vi "LeapMain.vi"() -> ()   [LabVIEW 2017]
uses:
  LeapMotion/TypeDefs/SelectSign.ctl
  LeapMotion/TypeDefs/StateSelector.ctl
  MachineLearning/TypeDefs/Label Setting.ctl
  C:/Users/snordinh/Desktop/LEAP-sign-language-test/LEAP-sign-language-test/LeapMotion/Dynamic Libraries/LeapCSharp.NET4.5.dll
  LeapMotion/Dynamic Libraries/LeapCSharp.NET4.5.dll
  LeapMotion/LeapMotion.lvlib
  MachineLearning/MachineLearning.lvlib
panel:
  in  "Clear text":bool
  in  "Interpret hand sign":bool
  out "Interpreted text":string
  in  "Tab Control":T1(tab)
  out "Real-time plot":cluster{sgl[], sgl[]}[](graph)
  out "Detected hand sign":T2
  out "feature trend deployment":dbl[][](graph)
  out "predicted result":i32[][](graph)
  out "metrics":T3
  in  "Error In":errorcluster
  out "Error out":errorcluster
  in  "Trained ML model":path=path "C:/Users/snordinh/Desktop/LEAP-sign-language-test/LEAP-sign-language-test/MachineLearning/SubVIs/WithDan.json"
  in  "Save model as":path
  in  "Train model":bool
  out "Points left to log":i32
  in  "Start logging":bool
  out "File saved as":path
  in  "Write header":bool
  in  "Points per sign":i32=100
  out "feature trend training":dbl[][](graph)
  out "Left hand detected":bool
  out "Right hand detected":bool
  in  "Hand sign":T2
  in  "Stop Program":bool
  out "LEAP connected?":bool
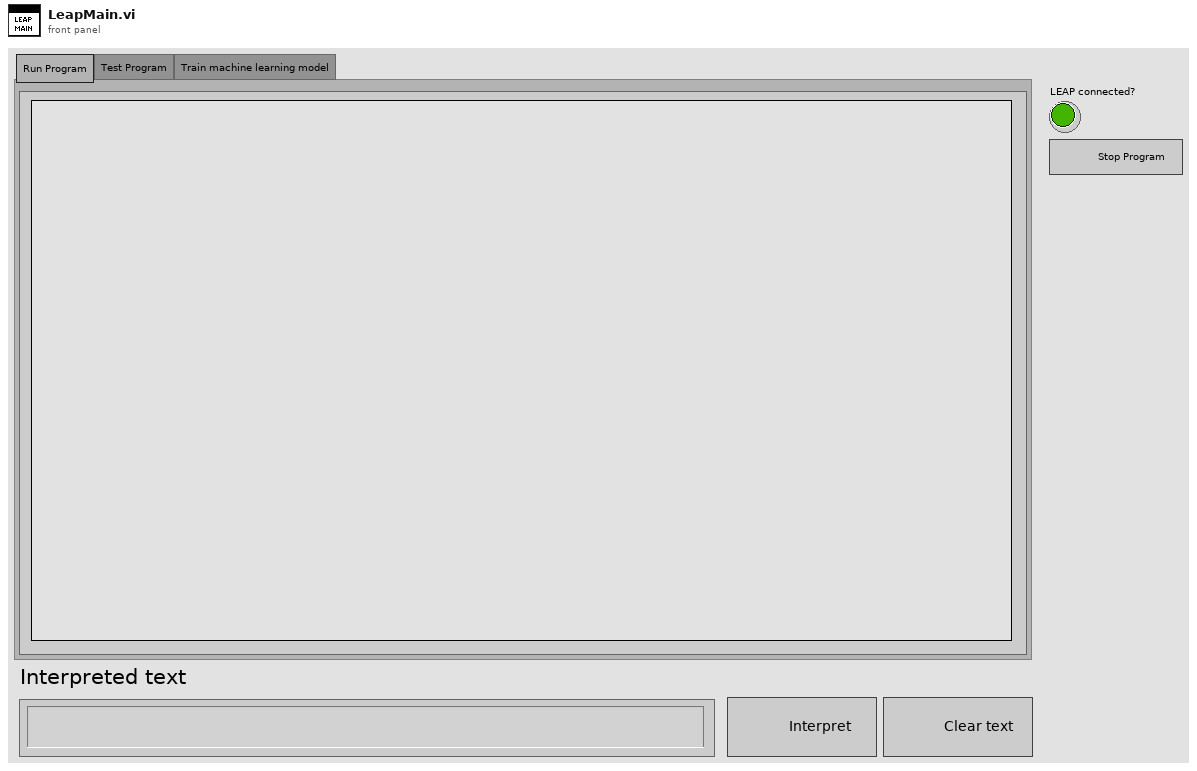
[diagram p1: front panel]
types:
  T1 = enum32{"Run Program", "Test Program", "Train machine learning model"}
  T2 = typedef "LeapMotion.lvlib/SelectSign.ctl" = enum16{"A", "B", "C", "D", "E", "F", "G", "H", "I", "J", "K", "L", "M", "N", "O", "P", "Q", "R", "S", "T", "U", "V", "W", "X", "Y", "Z"}
  T3 = cluster{"accuracy":dbl, "precision":dbl, "recall":dbl, "f1 score":dbl}
  T4 = typedef "LeapMotion.lvlib/StateSelector.ctl" = enum16{"Initialize", "Display", "Logging sequence", "Train model", "Classify", "Write Header", "Stop"}
  T5 = typedef "MachineLearning.lvlib/Label Setting.ctl" = cluster{"with label column?":bool, "label column index":i32}
  T6 = typedef "LeapMotion.lvlib/LEAPframe.ctl" = cluster{"Id":i64, "Timestamp":i64, "CurrentFramesPerSecond":sgl, "Hands":T7[]}
  T7 = typedef "LeapMotion.lvlib/LEAPhand.ctl" = cluster{"IsLeft":bool, "IsRight":bool, "Id":i32, "FrameId":i64, "Confidence":sgl, "TimeVisible":sgl, "PalmPosition":T8, "Fingers":T9[]}
  T8 = typedef "LeapMotion.lvlib/LEAPvector.ctl" = cluster{"Pitch":sgl, "Yaw":sgl, "Roll":sgl, "Magnitude":sgl, "XYZ":sgl[]}
  T9 = typedef "LeapMotion.lvlib/LEAPfinger.ctl" = cluster{"IsExtended":bool, "Id":i32, "Type":i32, "HandId":i32, "Length":sgl, "Width":sgl, "TimeVisible":sgl, "TipPosition":T8, "Bones":T10[]}
  T10 = typedef "LeapMotion.lvlib/LEAPbone.ctl" = cluster{"Type":i32, "Width":sgl, "Length":sgl, "Center":T8, "Direction":T8, "NextJoint":T8, "PrevJoint":T8}
  T11 = enum16{"SVM", "Neural Network", "Logistic Regression"}
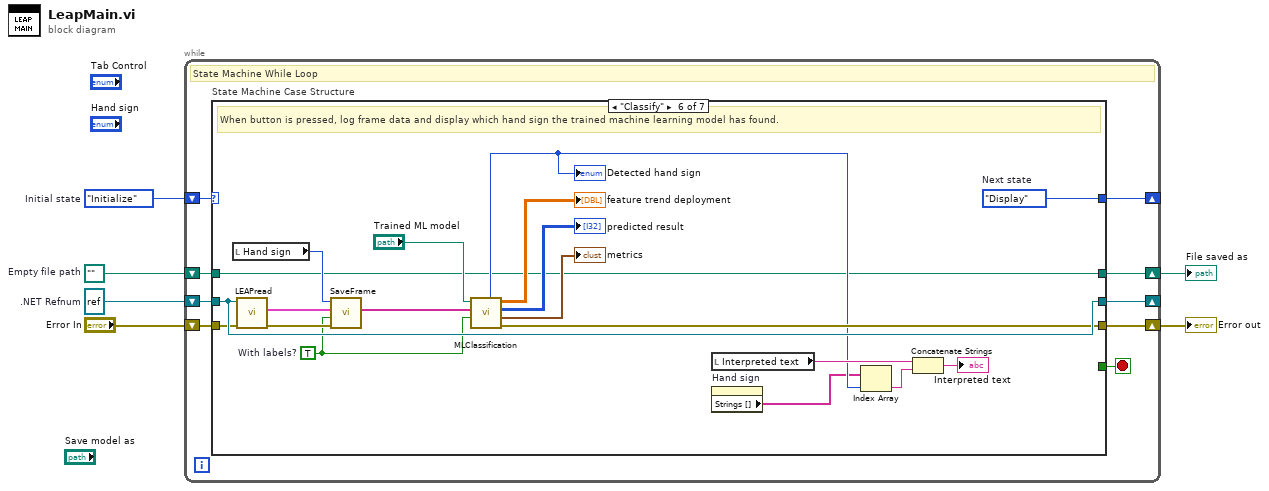
[diagram p0: block diagram]
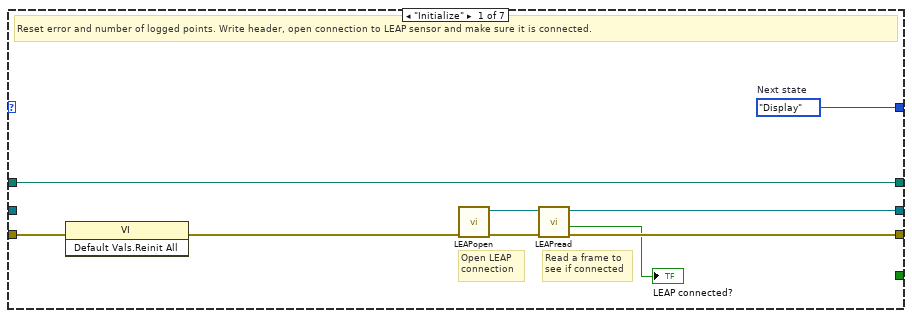
[diagram p2: hidden frame]
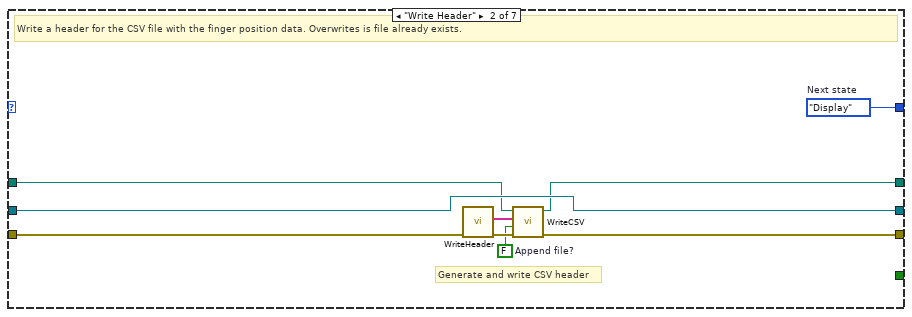
[diagram p3: hidden frame]
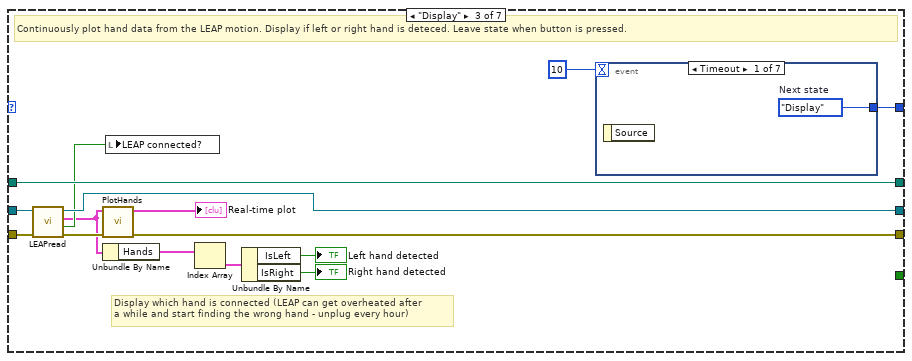
[diagram p4: hidden frame]
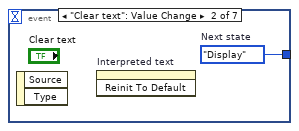
[diagram p5: hidden frame]
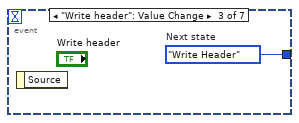
[diagram p6: hidden frame]
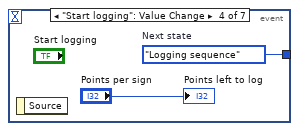
[diagram p7: hidden frame]
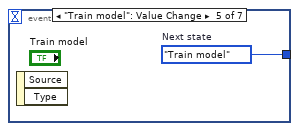
[diagram p8: hidden frame]
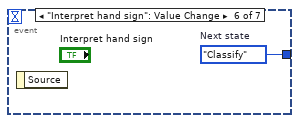
[diagram p9: hidden frame]
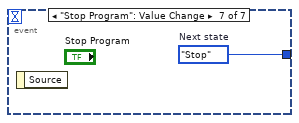
[diagram p10: hidden frame]
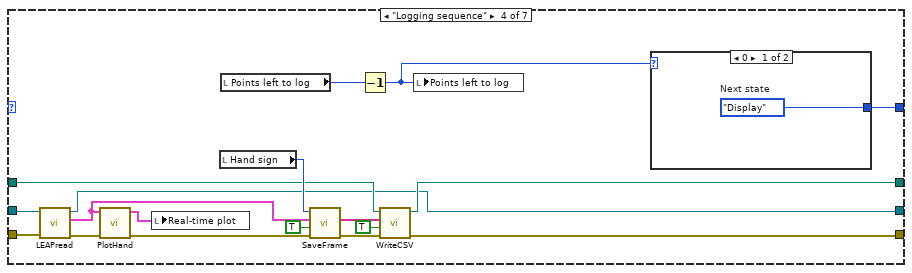
[diagram p11: hidden frame]
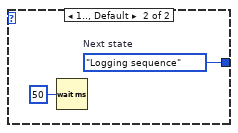
[diagram p12: hidden frame]
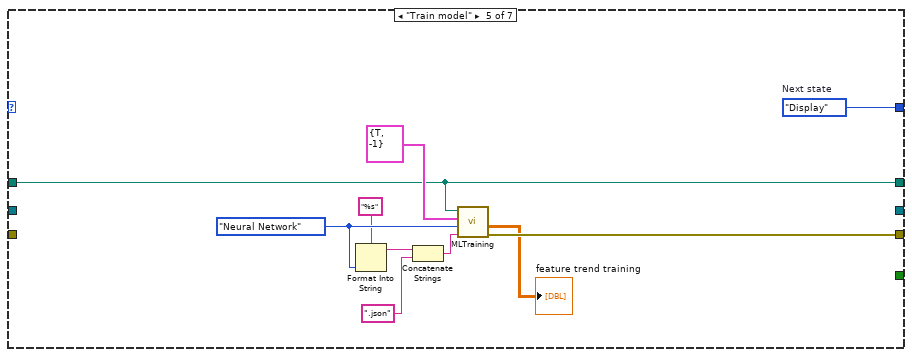
[diagram p13: hidden frame]
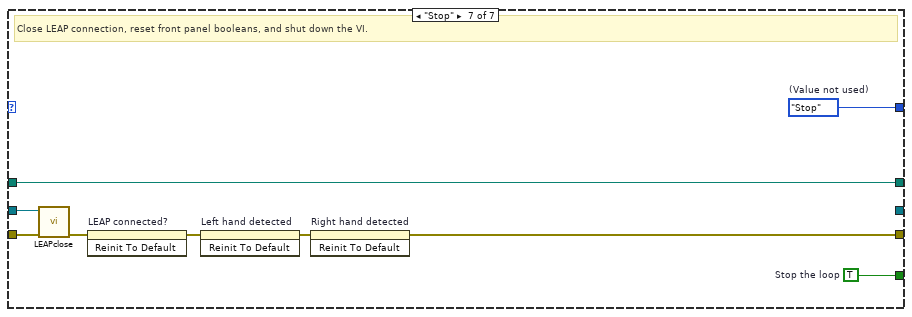
[diagram p14: hidden frame]
diagram:
  w4 = path ""  # Empty file path
  w2 = refnum<k24> refnum  # .NET Refnum
  w1 = StateSelector."Initialize"  # Initial state
  n1 = while {
    shift-right: [w15] -> _
    shift-left: w2 -> [w13]
    shift-right: [w14] -> w5
    shift-left: "Error In" -> [w12]
    shift-right: [w9] -> w3
    shift-left: w4 -> [w10]
    shift-right: [w7] -> _
    shift-left: w1 -> [w8]
    stop <- w11 stop-if-true
    # "State Machine While Loop"
    n2 = case "State Machine Case Structure" shown="\"Classify\"" w8 {
      tunnel: [_ _ _ _ _ _ w115] -> w11
      tunnel: [w17 w33 w40 w59 _ w103 _] -> w15
      tunnel: [w19 w27 w37 w60 w87 w96 w112] -> w14
      tunnel: w13 -> [_ w33 w42 w73 _ w103 w110]
      tunnel: w12 -> [w24 w32 w41 w74 _ w102 w109]
      tunnel: w10 -> [w23 w29 w43 w62 w84 w92 w111]
      tunnel: [w23 w28 w43 w61 w84 w92 w111] -> w9
      tunnel: [w16 w25 w34 w57 w79 w89 w107] -> w7
      frame "Initialize" {
        w16 = StateSelector."Display"  # Next state
        # "Read a frame to\nsee if connected"
        # "Open LEAP \nconnection"
        # "Reset error and number of logged points. Write header, open connection to LEAP sensor and make sure it is connected."
        n3 = invoke class="VI" method="Default Vals.Reinit All"(error in=w24) -> (error out=w22:errorcluster)  [unwired: 2 in, 2 out]
        n4 = call "LEAPopen.vi"("error in (no error)"=w22) -> ("error out"=w20:errorcluster, "Leap.Controller"=w21:refnum<k24>)  [unwired: 9 in]
        n5 = call "LEAPread.vi"("error in (no error)"=w20, "Controller Refnum In"=w21) -> ("error out"=w19:errorcluster, "IsConnected"=→"LEAP connected?":bool, "Leap.Controller"=w17:refnum<k24>)  [unwired: 6 in, 1 out]
      }
      frame "Write Header" {
        w26 = FALSE  # Append file?
        w25 = StateSelector."Display"  # Next state
        # "Generate and write CSV header"
        # "Write a header for the CSV file with the finger position data. Overwrites is file already exists."
        n6 = call "WriteHeader.vi"("Error in"=w32) -> ("Error out"=w31:errorcluster, "Header string array"=w30:string[])  [unwired: 9 in]
        n7 = call "WriteCSV.vi"("error in (no error)"=w31, "Append file?"=w26, "Data to write"=w30, "CSV file path in"=w29) -> ("error out"=w27:errorcluster, "CSV file path out"=w28:path)  [unwired: 6 in]
      }
      frame "Display" {
        # "Display which hand is connected (LEAP can get overheated after\na while and start finding the wrong hand - unplug every hour)"
        # "Continuously plot hand data from the LEAP motion. Display if left or right hand is deteced. Leave state when button is pressed."
        n8 = call "LEAPread.vi"("error in (no error)"=w41, "Controller Refnum In"=w42) -> ("error out"=w36:errorcluster, "IsConnected"=w39:bool, "Frame"=w35:T6, "Leap.Controller"=w40:refnum<k24>)  [unwired: 6 in]
        n9 = call "PlotHands.vi"("error in"=w36, "Frame"=w35) -> ("error out"=w37:errorcluster, "Data to plot"=→"Real-time plot":cluster{"Array":sgl[], "Array":sgl[]}[])  [unwired: 8 in]
        n10 = Unbundle By Name(w35) -> ("Hands"=w44:T7[])
        n11 = local write "LEAP connected?"(w39) -> ()
        n12 = Index Array(array=w44) -> (element=w45:T7)  [unwired: 1 in]
        n13 = Unbundle By Name(w45) -> ("IsLeft"=→"Left hand detected":bool, "IsRight"=→"Right hand detected":bool)
        n14 = event shown="[0] Timeout" {
          selector: _ -> [_ _ _ _ _ _ _]
          dyn-events: _ -> [_ _ _ _ _ _ _]
          timeout: 10 -> [_ _ _ _ _ _ _]
          tunnel: [w49 w50 w51 w53 w54 w55 w56] -> w34
          event Timeout {
            w49 = StateSelector."Display"  # Next state
            n15 = event-data() -> ()  [unwired: 1 in, 1 out]
          }
          event "Clear text": Value Change {
            w50 = StateSelector."Display"  # Next state
            n16 = event-data() -> ()  [unwired: 1 in, 2 out]
            n17 = invoke on="Interpreted text" class="Str" method="Reinit To Default"() -> ()  [unwired: 3 in, 3 out]
          }
          event "Write header": Value Change {
            w51 = StateSelector."Write Header"  # Next state
            n18 = event-data() -> ()  [unwired: 1 in, 1 out]
          }
          event "Start logging": Value Change {
            w53 = StateSelector."Logging sequence"  # Next state
            n19 = event-data() -> ()  [unwired: 1 in, 1 out]
            "Points left to log" <- "Points per sign"
          }
          event "Train model": Value Change {
            w54 = StateSelector."Train model"  # Next state
            n20 = event-data() -> ()  [unwired: 1 in, 2 out]
          }
          event "Interpret hand sign": Value Change {
            w55 = StateSelector."Classify"  # Next state
            n21 = event-data() -> ()  [unwired: 1 in, 1 out]
          }
          event "Stop Program": Value Change {
            w56 = StateSelector."Stop"  # Next state
            n22 = event-data() -> ()  [unwired: 1 in, 1 out]
          }
        }
      }
      frame "Logging sequence" {
        n23 = call "LEAPread.vi"("error in (no error)"=w74, "Controller Refnum In"=w73) -> ("error out"=w72:errorcluster, "Frame"=w67:T6, "Leap.Controller"=w59:refnum<k24>)  [unwired: 6 in, 1 out]
        n24 = call "PlotHand.vi"("error in"=w72, "Frame"=w67) -> ("error out"=w71:errorcluster, "Data to plot"=w68:cluster{"Array":sgl[], "Array":sgl[]}[])  [unwired: 8 in]
        n25 = local write "Real-time plot"(w68) -> ()
        n26 = local read "Hand sign"() -> (w69:T2)
        n27 = local read "Points left to log"() -> (w64:i32)
        n28 = call "SaveFrame.vi"("Error In"=w71, "With labels?"=TRUE, "Frame"=w67, "Hand sign"=w69) -> ("Error Out"=w70:errorcluster, "Frame data"=w66:string[])  [unwired: 6 in]
        n29 = Decrement(x=w64) -> (x-1=w58:i32)
        n30 = call "WriteCSV.vi"("error in (no error)"=w70, "Append file?"=TRUE, "Data to write"=w66, "CSV file path in"=w62) -> ("error out"=w60:errorcluster, "CSV file path out"=w61:path)  [unwired: 6 in]
        n31 = local write "Points left to log"(w58) -> ()
        n32 = case shown="0" w58 {
          tunnel: [w75 w77] -> w57
          frame 0 {
            w75 = StateSelector."Display"  # Next state
          }
          frame 1.., Default {
            w77 = StateSelector."Logging sequence"  # Next state
            n33 = Wait (ms)(milliseconds to wait=u32 50) -> ()  [unwired: 1 out]
          }
        }
      }
      frame "Train model" {
        w82 = T11."Neural Network" ("model to train")
        w79 = StateSelector."Display"  # Next state
        n34 = Format Into String(format string="%s", w82) -> (resulting string=w81:string)  [unwired: 2 in, 1 out]
        n35 = Concatenate Strings(w81, ".json" ("string")) -> (w83:string)
        n36 = call "MLTraining.vi"("Save model file as"=w83, "model to train"=w82, "Label setting"=T5 {"with label column?"=TRUE, "label column index"=-1}, "training data file (CSV)"=w84) -> ("error out"=w87:errorcluster, "feature trend"=→"feature trend training":dbl[][])  [unwired: 6 in]
      }
      frame "Classify" {
        w91 = TRUE  # With labels?
        w89 = StateSelector."Display"  # Next state
        # "When button is pressed, log frame data and display which hand sign the trained machine learning model has found."
        n37 = local read "Hand sign"() -> (w93:T2)
        n38 = call "LEAPread.vi"("error in (no error)"=w102, "Controller Refnum In"=w103) -> ("error out"=w101:errorcluster, "Frame"=w100:T6)  [unwired: 6 in, 2 out]
        n39 = call "SaveFrame.vi"("Error In"=w101, "With labels?"=w91, "Frame"=w100, "Hand sign"=w93) -> ("Frame data"=w90:string[])  [unwired: 6 in, 1 out]
        n40 = call "MLClassification.vi"("with labels?"=w91, "Frame data"=w90, "model file (JSON)"="Trained ML model") -> ("error out"=w96:errorcluster, "metrics"=→"metrics":T3, "predicted result"=→"predicted result":i32[][], "feature trend"=→"feature trend deployment":dbl[][], "Detected hand sign"=w94:i32)  [unwired: 4 in]
        "Detected hand sign" <- w94
        n41 = local read "Interpreted text"() -> (w106:string)
        n42 = property on="Hand sign" class="Enum (strict)"() -> ("Strings []"=w88:string[])  [unwired: 2 in, 2 out]
        n43 = Index Array(array=w88, index=w94) -> (element=w104:string)
        n44 = Concatenate Strings(w106, w104) -> (→"Interpreted text":string)
      }
      frame "Stop" {
        w115 = TRUE  # Stop the loop
        w107 = StateSelector."Stop"  # (Value not used)
        # "Close LEAP connection, reset front panel booleans, and shut down the VI."
        n45 = call "LEAPclose.vi"("error in (no error)"=w109, ".NET Refnum in"=w110) -> ("error out"=w108:errorcluster)  [unwired: 9 in]
        n46 = invoke on="LEAP connected?" class="Bool (strict)" method="Reinit To Default"(error in=w108) -> (error out=w114:errorcluster)  [unwired: 2 in, 2 out]
        n47 = invoke on="Left hand detected" class="Bool (strict)" method="Reinit To Default"(error in=w114) -> (error out=w113:errorcluster)  [unwired: 2 in, 2 out]
        n48 = invoke on="Right hand detected" class="Bool (strict)" method="Reinit To Default"(error in=w113) -> (error out=w112:errorcluster)  [unwired: 2 in, 2 out]
      }
    }
  }
  "Error out" <- w5
  "File saved as" <- w3
